vi "Calc Inputs.vi"(8 "error in (no error)":errorcluster, 11 "Min Calc in":refnum<class "Min Calc.lvclass">) -> (0 "error out":errorcluster, 2 "Inputs":string[](array[string]))   [LabVIEW 2020, in "VolatusCalcs.lvlib" / "Min Calc.lvclass"]
uses:
  Min Calc.lvclass
  Min Calc.lvclass/Min Calc.ctl
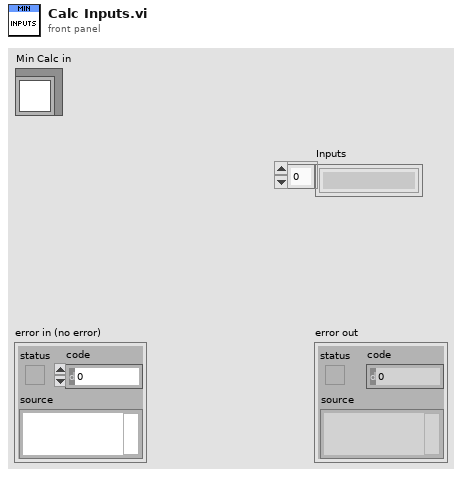
[diagram p1: front panel]
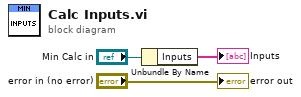
[diagram p0: block diagram]
diagram:
  n1 = Unbundle By Name("Min Calc in") -> ("Inputs"=→"Inputs":string[])
  "error out" <- "error in (no error)"
